vi "Get SMO Database Paths.vi"(5 "getAll Cluster":variant, 7 "Default Paths":string, 8 "error in (no error)":errorcluster, 11 "instrument.Cryostation in":refnum<class "instrument.Cryostation.lvclass">) -> (0 "error out":errorcluster, 2 "Paths":string, 3 "instrument.Cryostation out":refnum<class "instrument.Cryostation.lvclass">)   [LabVIEW 2019, in "instrument.Cryostation.lvclass"]
uses:
  instrument.Cryostation.lvclass
  Typedefs/Cryostation.getAll--cluster.ctl
  <userlib>/LevyLab/Instrument Framework/Instrument Types/Cryostat/Instrument.Cryostat.lvclass
  <userlib>/LevyLab/LV-Data/LV-Data.PG/LV-Data.PGSQL.lvclass
  <userlib>/LevyLab/LV-Data/LV-Data.PG/API/Write Variable (one-row).vi
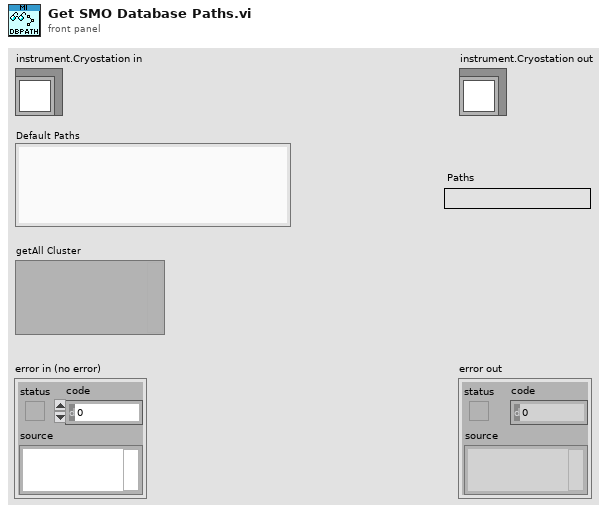
[diagram p1: front panel]
types:
  T1 = typedef "instrument.Cryostation.lvclass/Cryostation.getAll--cluster.ctl" = cluster{"Chamber Pressure (mTorr)":dbl, "Compressor Return Pressure (MPa)":dbl, "Compressor Supply Pressure (MPa)":dbl, "Compressor Speed (Hz)":dbl, "Cold Head Speed (Hz)":dbl, "Platform Heater Power (W)":dbl, "Platform Stability (K)":dbl, "Platform Temperature (K)":dbl, "Stage 1 Heater Power (W)":dbl, "Stage 1 Temperature (K)":dbl, "Stage 2 Heater Power (W)":dbl, "Stage 2 Temperature (K)":dbl, "Sample Stability (K)":dbl, "Sample Temperature (K)":dbl, "Temperature Set Point (K)":dbl, "User Stability (K)":dbl, "User Temperature (K)":dbl, "User Temperature Set Point (K)":dbl, "Alarm State":string, "Compressor Run State":string, "Case Valve State":string, "Idle State":string, "Nitrogen State":string, "Vent Valve State":string}
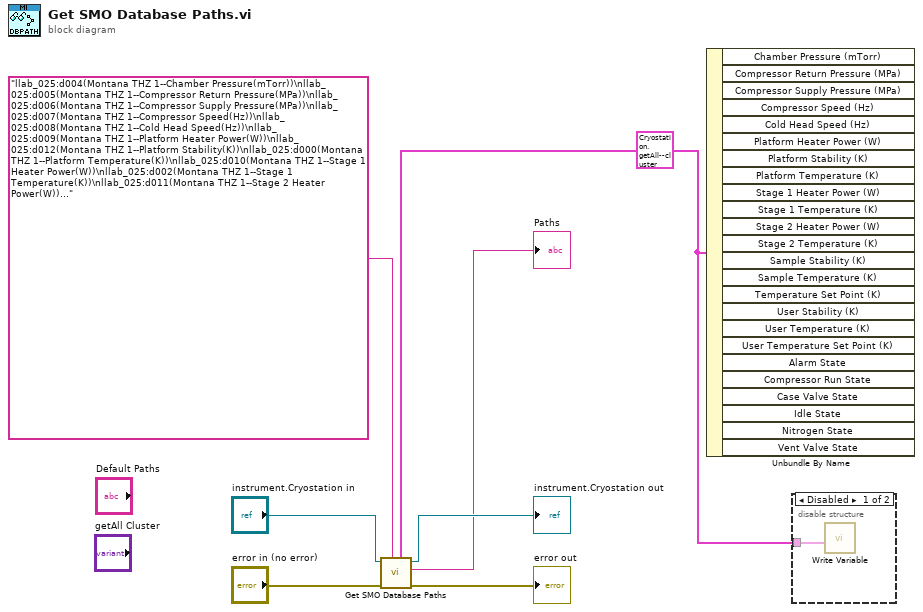
[diagram p0: block diagram]
diagram:
  w2 = T1 {"Chamber Pressure (mTorr)"=0.0, "Compressor Return Pressure (MPa)"=0.0, "Compressor Supply Pressure (MPa)"=0.0, "Compressor Speed (Hz)"=0.0, "Cold Head Speed (Hz)"=0.0, "Platform Heater Power (W)"=0.0, "Platform Stability (K)"=0.0, "Platform Temperature (K)"=0.0, "Stage 1 Heater Power (W)"=0.0, "Stage 1 Temperature (K)"=0.0, "Stage 2 Heater Power (W)"=0.0, "Stage 2 Temperature (K)"=0.0, "Sample Stability (K)"=0.0, "Sample Temperature (K)"=0.0, "Temperature Set Point (K)"=0.0, "User Stability (K)"=0.0, "User Temperature (K)"=0.0, "User Temperature Set Point (K)"=0.0, "Alarm State"="", "Compressor Run State"="", "Case Valve State"="", "Idle State"="", "Nitrogen State"="", "Vent Valve State"=""} ("getAll")
  n1 = call-parent "Get SMO Database Paths.vi"("getAll Cluster"=w2, "Default Paths"="llab_025:d004(Montana THZ 1--Chamber Pressure(mTorr))\nllab_025:d005(Montana THZ 1--Compressor Return Pressure(MPa))\nllab_025:d006(Montana THZ 1--Compressor Supply Pressure(MPa))\nllab_025:d007(Montana THZ 1--Compressor Speed(Hz))\nllab_025:d008(Montana THZ 1--Cold Head Speed(Hz))\nllab_025:d009(Montana THZ 1--Platform Heater Power(W))\nllab_025:d012(Montana THZ 1--Platform Stability(K))\nllab_025:d000(Montana THZ 1--Platform Temperature(K))\nllab_025:d010(Montana THZ 1--Stage 1 Heater Power(W))\nllab_025:d002(Montana THZ 1--Stage 1 Temperature(K))\nllab_025:d011(Montana THZ 1--Stage 2 Heater Power(W))\nllab_025:d003(Montana THZ 1--Stage 2 Temperature(K))\nllab_025:d013(Montana THZ 1--Sample Stability(K))\nllab_025:d001(Montana THZ 1--Sample Temperature(K))\nllab_025:d014(Montana THZ 1--Temperature Set Point(K))\nllab_025:d015(Montana THZ 1--User Stability(K))\nllab_025:d016(Montana THZ 1--User Temperature(K))\nllab_025:d017(Montana THZ 1--User Temperature Set Point(K))\nllab_025:v002(Montana THZ 1--Alarm State())\nllab_025:v003(Montana THZ 1--Compressor Run State())\nllab_025:v004(Montana THZ 1--Case Valve State())\nllab_025:v005(Montana THZ 1--Idle State())\nllab_025:v006(Montana THZ 1--Nitrogen State())\nllab_025:v007(Montana THZ 1--Vent Valve State())" ("Paths"), "error in (no error)"="error in (no error)", "Instrument in"="instrument.Cryostation in") -> ("error out"=→"error out":errorcluster, "Paths"=→"Paths":string, "Instrument out"=→"instrument.Cryostation out":refnum<class "instrument.Cryostation.lvclass">)  [unwired: 5 in]
  n2 = Unbundle By Name(w2) -> ()  [unwired: 24 out]
  n3 = disable-structure shown="Disabled" {
    disable-tunnel: w2 -> [w8 _]
    frame Disabled {
      n4 = call-poly <userlib>:"Write Variable.vi"("Data"=w8) -> ()  [unwired: 7 in, 4 out]
    }
    frame Enabled {
    }
  }
